vi "Flatten Linked List.vi"(6 "Persistence":refnum<class "IPersist.lvclass">, 7 "Linked List ID":string, 8 "error in (no error)":errorcluster, 11 "Linked List Ref":refnum<data-value>) -> (0 "error out":errorcluster, 2 "Flattened Linked List":string, 3 "Linked List Ref out":refnum<data-value>)   [LabVIEW 2020, in "Linked Lists.lvlib" / "Linked List Ref.lvclass"]
uses:
  <vilib>/gpm_packages/@cs/linked-list/Source/Linked List/Linked List Ref/Linked List Ref.lvclass
  <vilib>/gpm_packages/@cs/linked-list/Source/Linked List/ILinkedList/ILinked List.lvclass
  <vilib>/gpm_packages/@cs/persistence/source/IPersist/IPersist.lvclass
  <vilib>/gpm_packages/@cs/linked-list/Source/String Manipulation/String Manipulation.lvlib
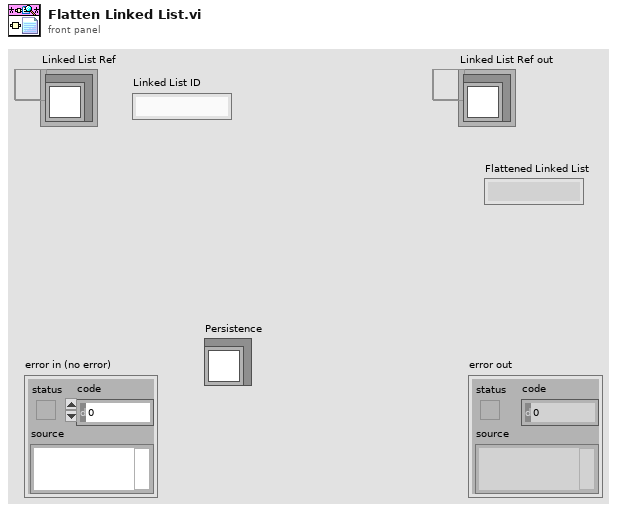
[diagram p1: front panel]
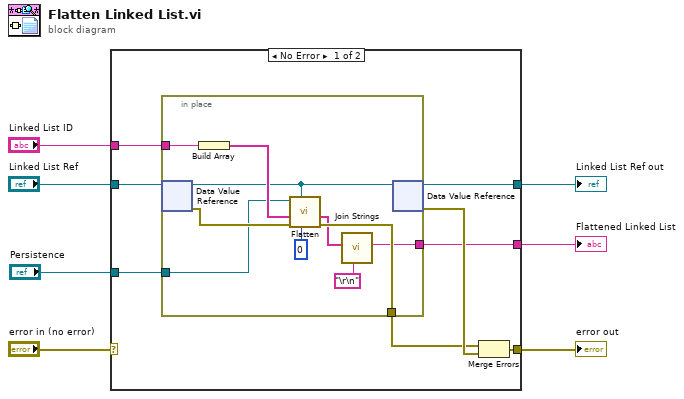
[diagram p0: block diagram]
diagram:
  n1 = case shown="No Error" "error in (no error)" {
    selector: "error in (no error)" -> [_ w27]
    tunnel: "Linked List Ref" -> [w15 w26]
    tunnel: "Linked List ID" -> [w14 _]
    tunnel: [w12 w27] -> w4
    tunnel: [w13 w26] -> w3
    tunnel: [w9 _] -> w2
    tunnel: "Persistence" -> [w8 _]
    frame No Error {
      n2 = in-place {
        in-place-border: w14 -> [w25]
        in-place-border: [w20] -> w10
        in-place-border: [w18] -> w9
        in-place-border: w8 -> [w16]
        n3 = in-place-dvr #1(w15) -> (w17:refnum<class "ILinked List.lvclass">, w22:errorcluster)
        n4 = Build Array(w25) -> (w24:string[])
        n5 = call-dynamic "Flatten.vi"("Indent"=0, "ILinked List in"=w17, "error in (no error)"=w22, "Child IDs"=w24, "IPersist in"=w16) -> ("error out"=w20:errorcluster, "Flattened Linked List"=w19:string[])  [unwired: 3 in, 2 out]
        n6 = call <vilib>:"Join Strings.vi"("Separator (,)"="\r\n", "Strings In"=w19) -> ("String"=w18:string)  [unwired: 9 in]
        n7 = in-place-dvr #1(w17) -> (w13:refnum<data-value>, w11:errorcluster)
      }
      n8 = Merge Errors(w10, w11) -> (w12:errorcluster)
    }
    frame Error {
    }
  }
  "error out" <- w4
  "Linked List Ref out" <- w3
  "Flattened Linked List" <- w2
